vi "Do.vi"(8 "error in (no error)":errorcluster, 9 "Events":refnum<class "Events.lvclass">, 10 "Message Loop Data in":T1, 11 "IInternalRequest in":refnum<class "HandleSubscribed JSON.lvclass">) -> (0 "error out":errorcluster, 2 "Message Loop Data out":T1, 3 "IInternalRequest out":refnum<class "HandleSubscribed JSON.lvclass">)   [LabVIEW 2020, in "wamplv.lvlib" / "HandleSubscribed JSON.lvclass"]
uses:
  HandleSubscribed JSON.lvclass
  HandleSubscribed JSON.lvclass/HandleSubscribed JSON.ctl
  SerialisedMessages/JSONMessage/WampMessage JSON.lvclass
  Message loop classes/Subscription details/SubscriptionDetails JSON/SubscriptionDetails JSON.lvclass
  Message loop classes/ErrorOrSuccess JSON/ErrorOrSuccess JSON.lvclass
  Error/ErrorHandler JSON/ErrorHandler JSON.lvclass
  Subscribe/ISubscribe/ISubscribe.lvclass
  <vilib>/ErrorRing/Error Ring.xnode
  <vilib>/Utility/error.llb/Error Cluster From Error Code.vi
  Public/Subscribe Result/SubscribeResult JSON/SubscribeResult JSON.lvclass
  C:/local/wamplv/Private/Message loop classes/Subscription details/SubscriptionDetailsParent/SubscriptionDetailsParent.lvclass
  C:/local/wamplv/Private/Requests/IContainersNotiferOrEvents/IContainersNotiferOrEvents.lvclass
  C:/local/wamplv/Private/Message loop classes/Subscription details/SubscriptionDetails JSON/SubscriptionDetails JSON.lvclass
  C:/local/wamplv/Public/Subscribe Result/ISubscribeResult/ISubscribeResult.lvclass
  C:/local/wamplv/Private/Message loop classes/IRequestResult/IRequestResult.lvclass
  C:/local/wamplv/Public/Subscribe Result/SubscribeResult JSON/SubscribeResult JSON.lvclass
  WAMP Client/Private/TypeDef/Publish Requests Map.ctl
  wamplv.lvlib
  WAMP Client/Private/TypeDef/Endpoint Data.ctl
  Call/ICallRequest/ICallRequest.lvclass
  WAMP Client/Private/TypeDef/CALL Request Map.ctl
  WAMP Client/Private/TypeDef/SUBSCRIBE Requests Map.ctl
  WAMP Client/Private/TypeDef/Subscriptions Map.ctl
  WAMP Client/Private/TypeDef/Unsubscribe Requests Map.ctl
  WAMP Client/Private/TypeDef/Unregister requests map.ctl
  WAMP Client/Private/TypeDef/Message Loop Data.ctl
  Events/EventsParent/Events.lvclass
  Publish/IPublish/IPublish.lvclass
  Message loop classes/Subscription details/SubscriptionDetailsParent/SubscriptionDetailsParent.lvclass
  Unsubscribe/IUnsubscribe/IUnsubscribe.lvclass
  Register/IRegister/IRegister.lvclass
  Unregister/IUnregister/IUnregister.lvclass
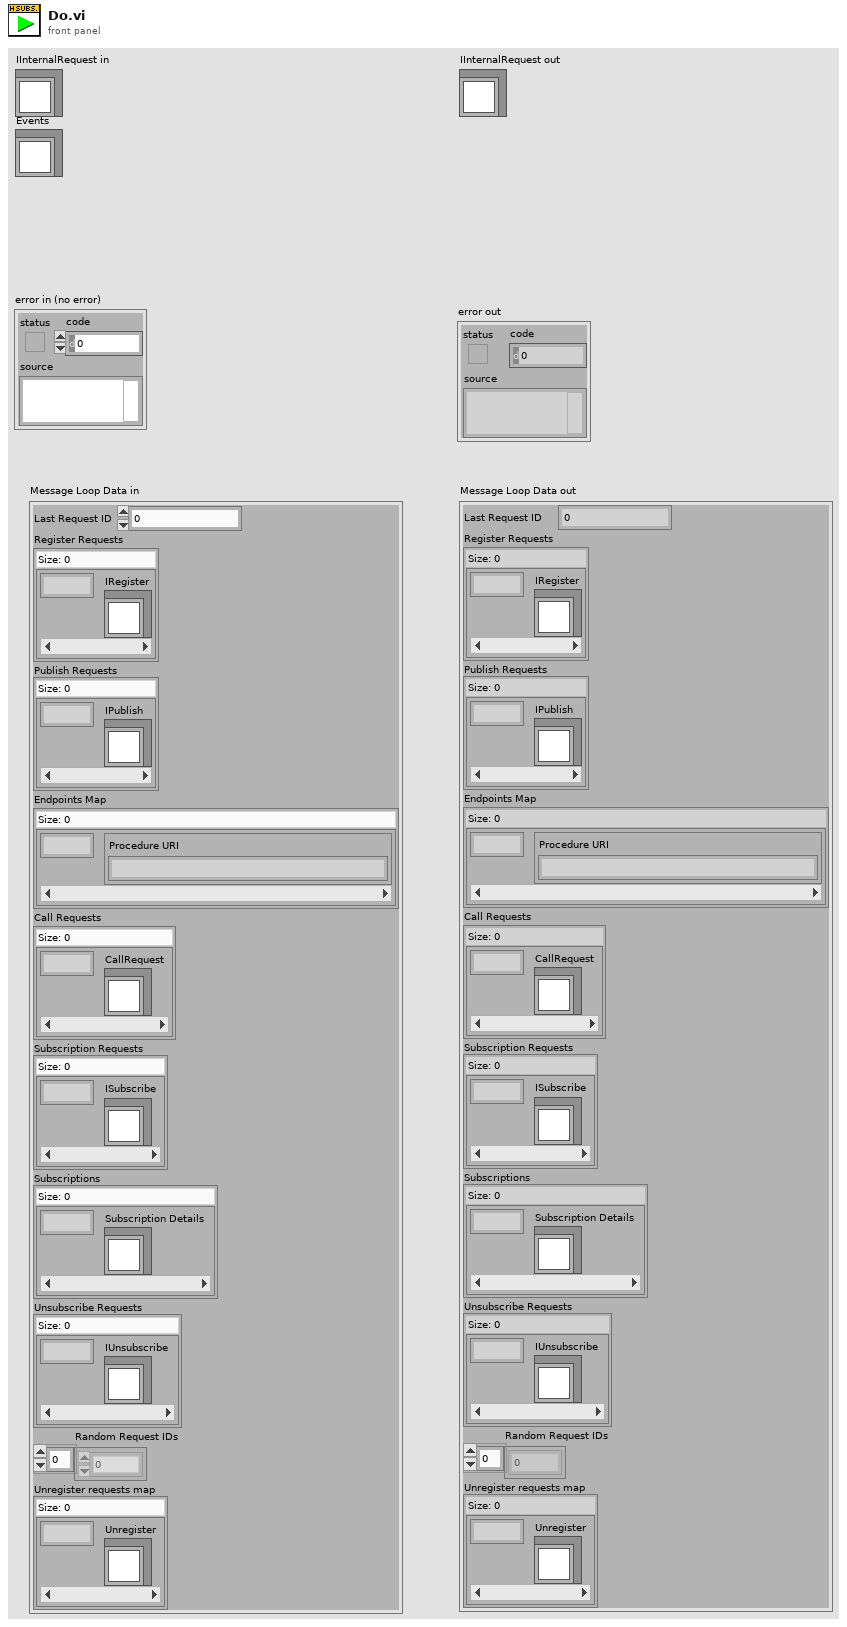
[diagram p1: front panel]
types:
  T1 = typedef "wamplv.lvlib/Message Loop Data.ctl" = cluster{"Last Request ID":u64, "Register Requests":map{u64, refnum<class "IRegister.lvclass">}, "Publish Requests":T2, "Endpoints Map":map{u64, T3}, "Call Requests":T4, "Subscription Requests":T5, "Subscriptions":T6, "Unsubscribe Requests":T7, "Random Request IDs":u64[], "Unregister requests map":T8}
  T2 = typedef "wamplv.lvlib/Publish Requests Map.ctl" = map{u64, refnum<class "IPublish.lvclass">}
  T3 = typedef "wamplv.lvlib/Endpoint Data.ctl" = cluster{"Procedure URI":string}
  T4 = typedef "wamplv.lvlib/CALL Request Map.ctl" = map{u64, refnum<class "ICallRequest.lvclass">}
  T5 = typedef "wamplv.lvlib/SUBSCRIBE Requests Map.ctl" = map{u64, refnum<class "ISubscribe.lvclass">}
  T6 = typedef "wamplv.lvlib/Subscriptions Map.ctl" = map{u64, refnum<class "SubscriptionDetailsParent.lvclass">}
  T7 = typedef "wamplv.lvlib/Unsubscribe Requests Map.ctl" = map{u64, refnum<class "IUnsubscribe.lvclass">}
  T8 = typedef "wamplv.lvlib/Unregister requests map.ctl" = map{u64, refnum<class "IUnregister.lvclass">}
  T9 = typedef "wamplv.lvlib/WAMP Message Codes.ctl" = enum8{"HELLO", "WELCOME", "CHALLENGE", "AUTHENTICATE", "ABORT", "GOODBYE", "ERROR", "PUBLISH", "PUBLISHED", "SUBSCRIBE", "SUBSCRIBED", "UNSUBSCRIBE", "UNSUBSCRIBED", "EVENT", "CALL", "RESULT", "REGISTER", "REGISTERED", "UNREGISTER", "UNREGISTERED", "INVOCATION", "YIELD"}
  T10 = typedef "wamplv.lvlib/Error (JSON).ctl" = cluster{"Request ID":u64, "Message type that caused error":T9, "Error/Abort details (JSON)":T11}
  T11 = typedef "wamplv.lvlib/Error or abort detail (JSON).ctl" = cluster{"Error URI":string, "Error Arguments":string, "Error ArgumentKw":string, "Error Details":string, "Associated LabVIEW Error":errorcluster}
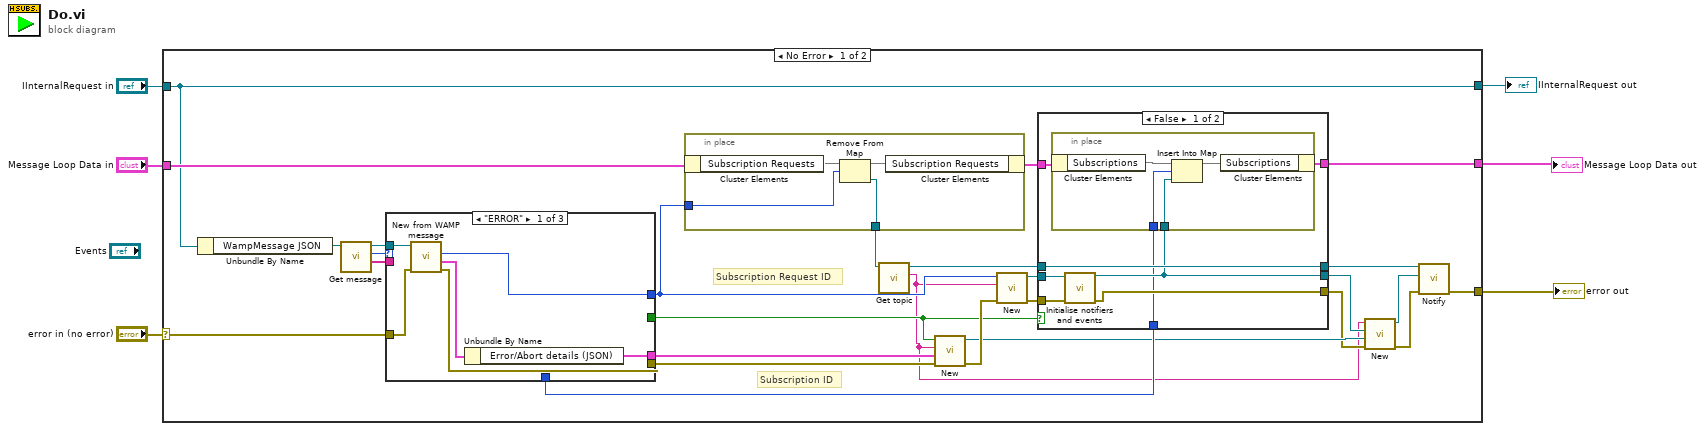
[diagram p0: block diagram]
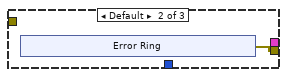
[diagram p2: hidden frame]
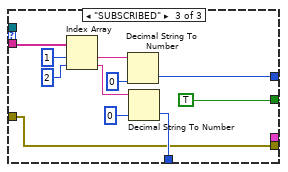
[diagram p3: hidden frame]
diagram:
  n1 = case shown="No Error" "error in (no error)" {
    selector: "error in (no error)" -> [w17 w77]
    tunnel: "Message Loop Data in" -> [w29 w76]
    tunnel: [w18 w76] -> w5
    tunnel: "IInternalRequest in" -> [w14 w78]
    tunnel: [w15 w77] -> w2
    tunnel: [w14 w78] -> w1
    frame No Error {
      # "Subscription ID"
      # "Subscription Request ID"
      n2 = Unbundle By Name(w14) -> ("WampMessage JSON"=w33:refnum<class "WampMessage JSON.lvclass">)
      n3 = call "Get message.vi"("JSONMessage in"=w33) -> ("<JSON>Elements"=w30:string[], "Message Type"=w32:T9, "JSONMessage out"=w31:refnum<class "WampMessage JSON.lvclass">)  [unwired: 8 in]
      n4 = case shown="\"ERROR\"" w32 {
        tunnel: w31 -> [w43 _ _]
        tunnel: w30 -> [_ _ w53]
        tunnel: [w42 _ w52] -> w27
        tunnel: [_ _ w51] -> w20
        tunnel: [_ _ TRUE] -> w21
        tunnel: [w40 _ _] -> w24
        tunnel: w17 -> [w39 _ w49]
        tunnel: [w38 w44 w49] -> w16
        frame "ERROR" {
          n5 = call "New from WAMP message.vi"("error in (no error)"=w39, "wamplv.lvlib:JSONMessage.lvclass"=w43) -> ("error out"=w38:errorcluster, "Error data (JSON)"=w41:T10, "Request ID"=w42:u64)  [unwired: 6 in, 1 out]
          n6 = Unbundle By Name(w41) -> ("Error/Abort details (JSON)"=w40:T11)
        }
        frame Default {
          n7 = xnode "Error Ring"() -> ("error out"=w44:errorcluster)
        }
        frame "SUBSCRIBED" {
          n8 = Index Array(array=w53, index #1=1 ("index"), index #2=2 ("index")) -> (element #1=w58:string, element #2=w54:string)
          n9 = Decimal String To Number(string=w58, default (0L)=u64 0) -> (number=w52:u64)  [unwired: 1 in, 1 out]
          n10 = Decimal String To Number(string=w54, default (0L)=u64 0) -> (number=w51:u64)  [unwired: 1 in, 1 out]
        }
      }
      n11 = in-place {
        in-place-border: w27 -> [w35]
        in-place-border: [w34] -> w28
        n12 = in-place-cluster #1(w29) -> ("Subscription Requests"=w36:T5)
        n13 = Remove From Map(10:w35, 11:w36) -> (1:w34:refnum<class "ISubscribe.lvclass">, 3:w37:T5)  [unwired: 1 out]
        n14 = in-place-cluster #1("Subscription Requests"=w37) -> (w19:T1)
      }
      n15 = call-dynamic "Get topic.vi"("ISubscribe in"=w28) -> ("Topic"=w7:string, "ISubscribe out"=w22:refnum<class "ISubscribe.lvclass">)  [unwired: 9 in]
      n16 = call "New.vi"("error in (no error)"=w16, "Error/Abort details (JSON)"=w24, "Request URI"=w7, "Success?"=w21) -> ("error out"=w23:errorcluster, "ErrorOrSuccess JSON out"=w13:refnum<class "ErrorOrSuccess JSON.lvclass">)  [unwired: 6 in]
      n17 = call "New.vi"("error in (no error)"=w23, "Topic"=w7, "Subscription ID"=w27) -> ("error out"=w26:errorcluster, "SubscriptionDetails JSON out"=w25:refnum<class "SubscriptionDetails JSON.lvclass">)  [unwired: 7 in]
      n18 = case shown="False" w21 {
        tunnel: w26 -> [w67 w75]
        tunnel: w25 -> [w66 w74]
        tunnel: [w65 w75] -> w11
        tunnel: [w63 w74] -> w10
        tunnel: w22 -> [w64 w73]
        tunnel: [w64 w73] -> w9
        tunnel: w20 -> [w62 _]
        tunnel: w19 -> [w61 w72]
        tunnel: [w60 w72] -> w18
        frame False {
          n19 = call-dynamic "Initialise notifiers and events.vi"("error in (no error)"=w67, "SubscriptionDetails JSON in"=w66) -> ("error out"=w65:errorcluster, "SubscriptionDetails JSON out"=w63:refnum<class "SubscriptionDetails JSON.lvclass">)  [unwired: 8 in]
          n20 = in-place {
            in-place-border: w63 -> [w70]
            in-place-border: w62 -> [w69]
            n21 = in-place-cluster #2(w61) -> ("Subscriptions"=w71:T6)
            n22 = Insert Into Map(map in=w71, key=w69, value=w70) -> (map out=w68:T6)  [unwired: 2 out]
            n23 = in-place-cluster #2("Subscriptions"=w68) -> (w60:T1)
          }
        }
        frame True {
        }
      }
      n24 = call "New.vi"("error in (no error)"=w11, "ErrorOrSuccess JSON"=w13, "SubscriptionDetails JSON"=w10, "Topic"=w7) -> ("error out"=w12:errorcluster, "SubscribeResult JSON out"=w8:refnum<class "SubscribeResult JSON.lvclass">)  [unwired: 6 in]
      n25 = call-dynamic "Notify.vi"("error in (no error)"=w12, "ISubscribeResult"=w8, "ISubscribe in"=w9) -> ("error out"=w15:errorcluster)  [unwired: 7 in, 1 out]
    }
    frame Error {
    }
  }
  "error out" <- w2
  "IInternalRequest out" <- w1
  "Message Loop Data out" <- w5
